vi "Trial - Editor.vi"(8 "Error IN":errorcluster) -> (0 "error out":errorcluster)   [LabVIEW 2018]
doc: "This VI allows the user to reprocess and reprint data sheets from previously run ESS test. User can search for vibe or thermal test for both actuators and controllers through this portal. Double click serial number from 'Available Data Files' listbox and press 'Print' to initiate report regeneration."
uses:
  controls/Trial Config Settings.ctl
  controls/Command IN_Recipe.ctl
  Globals/Global - Configuration Options.vi
panel:
  in  "Copy":bool
  in  "Trial Config Parameter Guide":bool
  in  "Rename":bool
  in  "Exit":bool
  out "Trial Name":string
  in  "Trial Settings":T1
  in  "Save":bool
  in  "New":bool
  in  "Delete":bool
  in  "Trial List":i32(listbox)
  in  "Refresh":bool
  out "Trial File Path":path
  in  "Functions":enum16{"Initialize", "Exit"}(ring)
  out "Trial Config Directory":path=path "C:/Data"
  # "Trial Configuration Screen"
  # "*click on trial file to view"
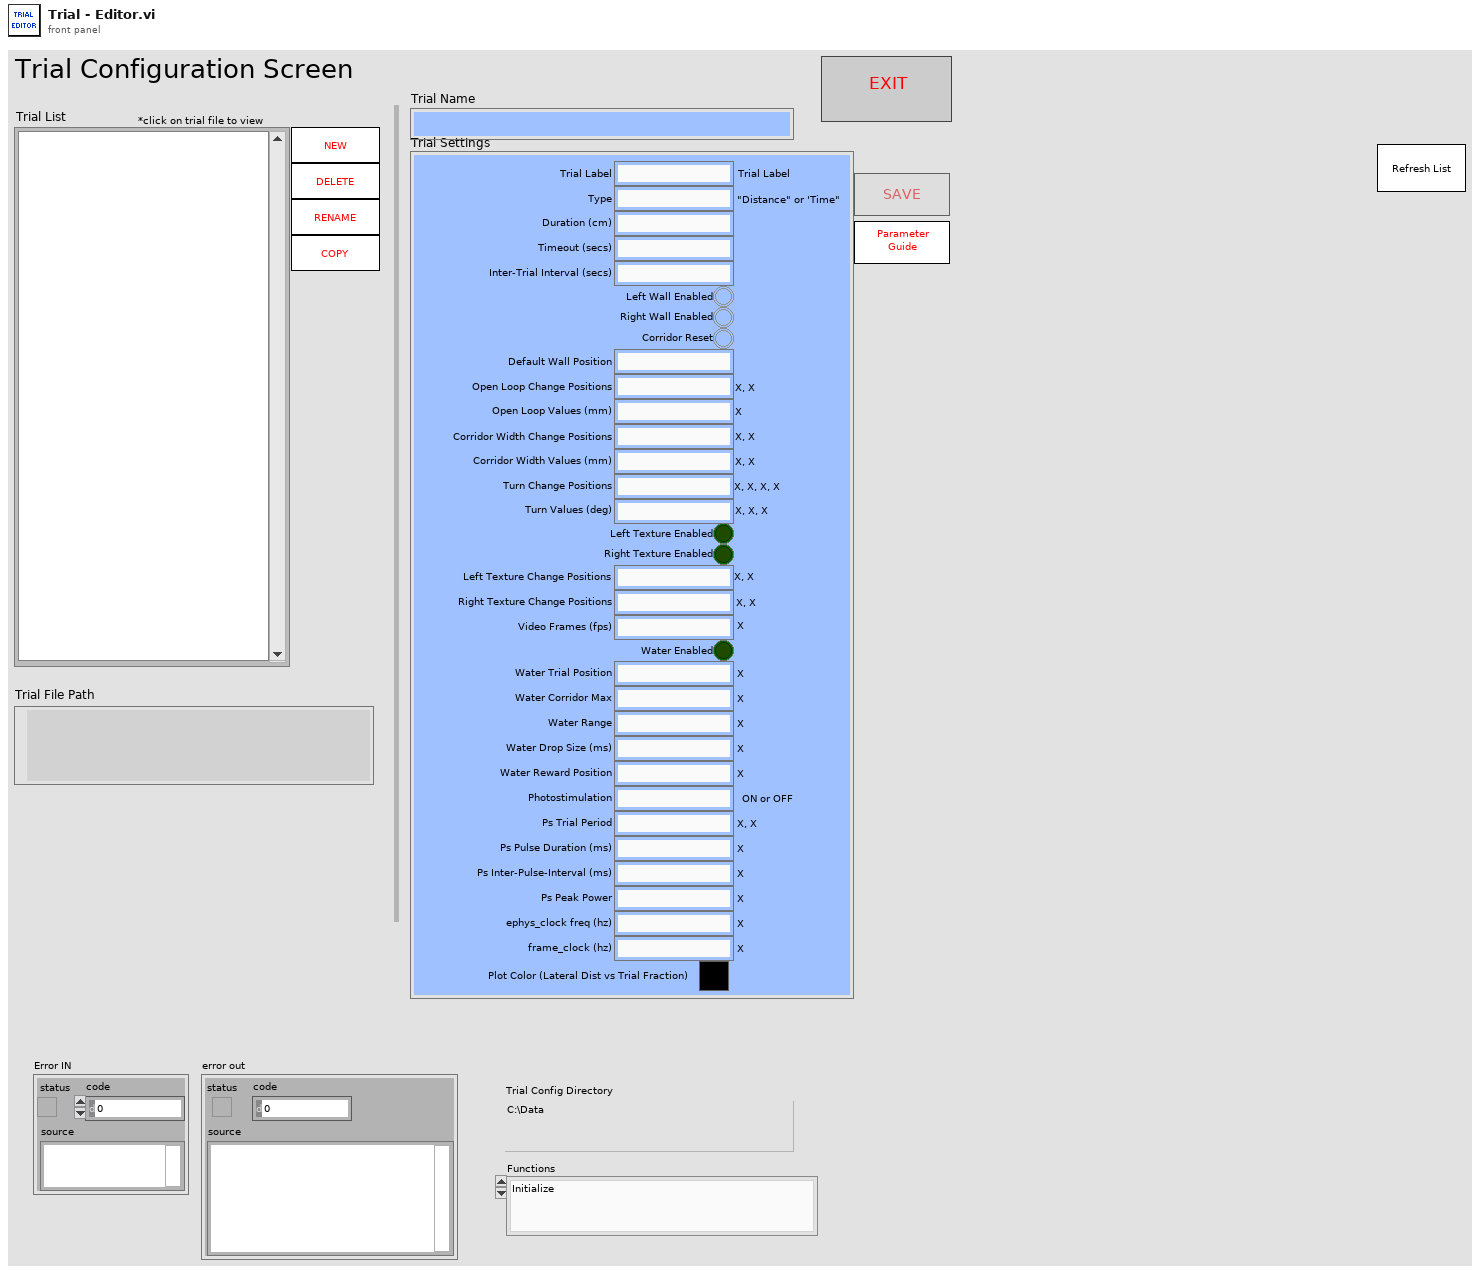
[diagram p1: front panel]
types:
  T1 = typedef "Trial Config Settings.ctl" = cluster{"Trial Label":string, "Type":string, "Timeout (secs)":string, "Inter-Trial Interval (secs)":string, "Left Wall Enabled":bool, "Right Wall Enabled":bool, "Corridor Reset":bool, "Default Wall Position":string, "Open Loop Change Positions":string, "Open Loop Values (mm)":string, "Corridor Width Change Positions":string, "Corridor Width Values (mm) ":string, "Turn Change Positions":string, "Turn Values (deg)":string, "Left Texture Change Positions":string, "Right Texture Change Positions":string, "Video Frames (fps)":string, "Water Enabled":bool, "Water Trial Position":string, "Photostimulation":string, "Water Corridor Max":string, "Water Range":string, "Water Drop Size (ms)":string, "Water Reward Position":string, "Duration (cm)":string, "Left Texture Enabled":bool, "Right Texture Enabled":bool, "Ps Trial Period":string, "Ps Inter-Pulse-Interval (ms)":string, "Ps Peak Power":string, "Ps Pulse Duration (ms)":string, "ephys_clock freq (hz)":string, "frame_clock (hz)":string, "Plot Color (Lateral Dist vs Trial Fraction)":u32}
  T2 = enum8{"Enabled", "Disabled", "Disabled and Grayed Out"}
  T3 = typedef "Command IN_Recipe.ctl" = enum16{"Save", "Load"}
  T4 = typedef "Rig Config Settings.ctl" = cluster{"Rig Name":string, "Rig Room":string, "Base Directory":string, "Computer IP Address":string, "Globals Name":string, "Treatmill Str":string, "cRIO Test Data Dir":path, "ai":string, "ao":string, "dio":string, "A_calib_str_row1":string, "A_calib_str_row2":string, "A_calib_str_row3":string, "Zero_V_str":string, "step_V":string, "Sample Freq":string, "ai_threshold":string, "run_speed_thresh":string, "speed_time_length":string, "wall ball gain":string, "max wall pos":string, "max cor width":string, "Trial Config Directory":path, "Randomize Trials?":bool}
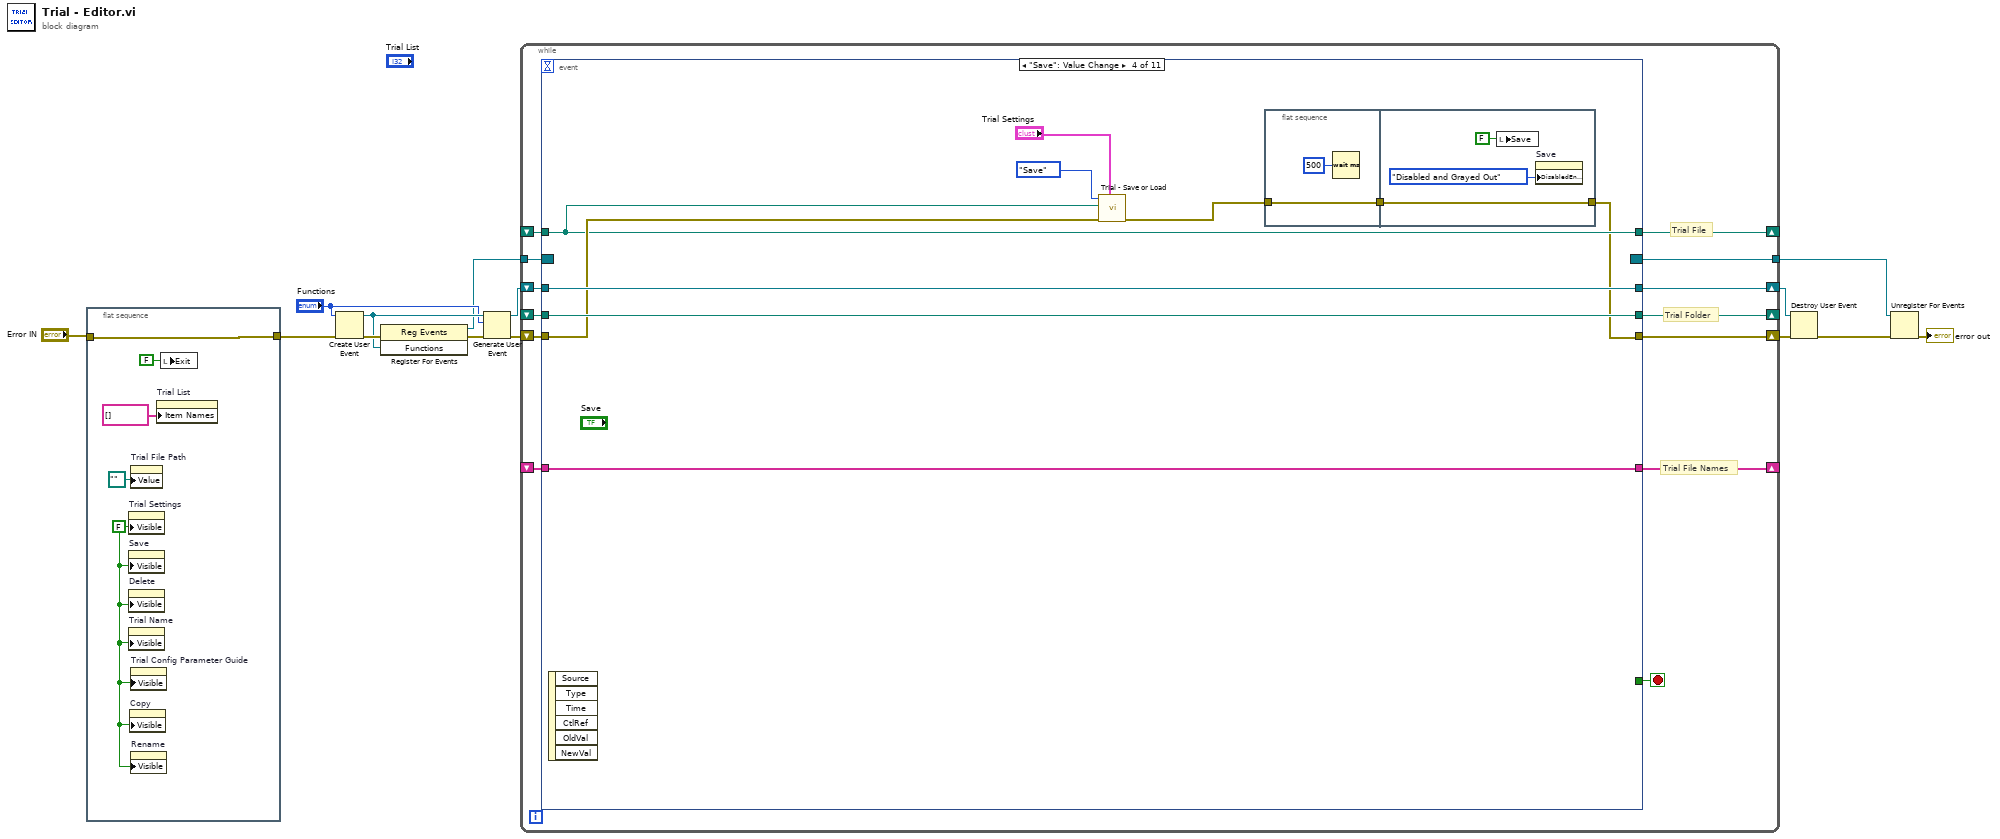
[diagram p0: block diagram]
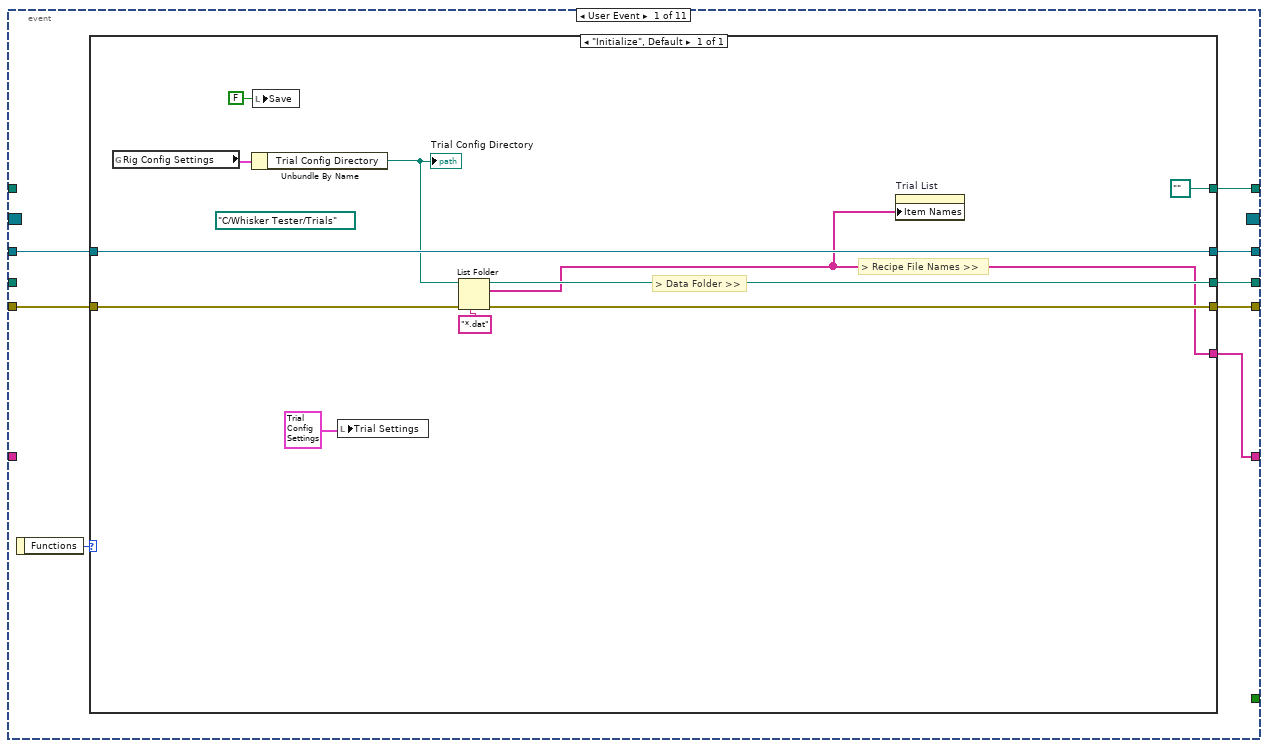
[diagram p2: hidden frame]
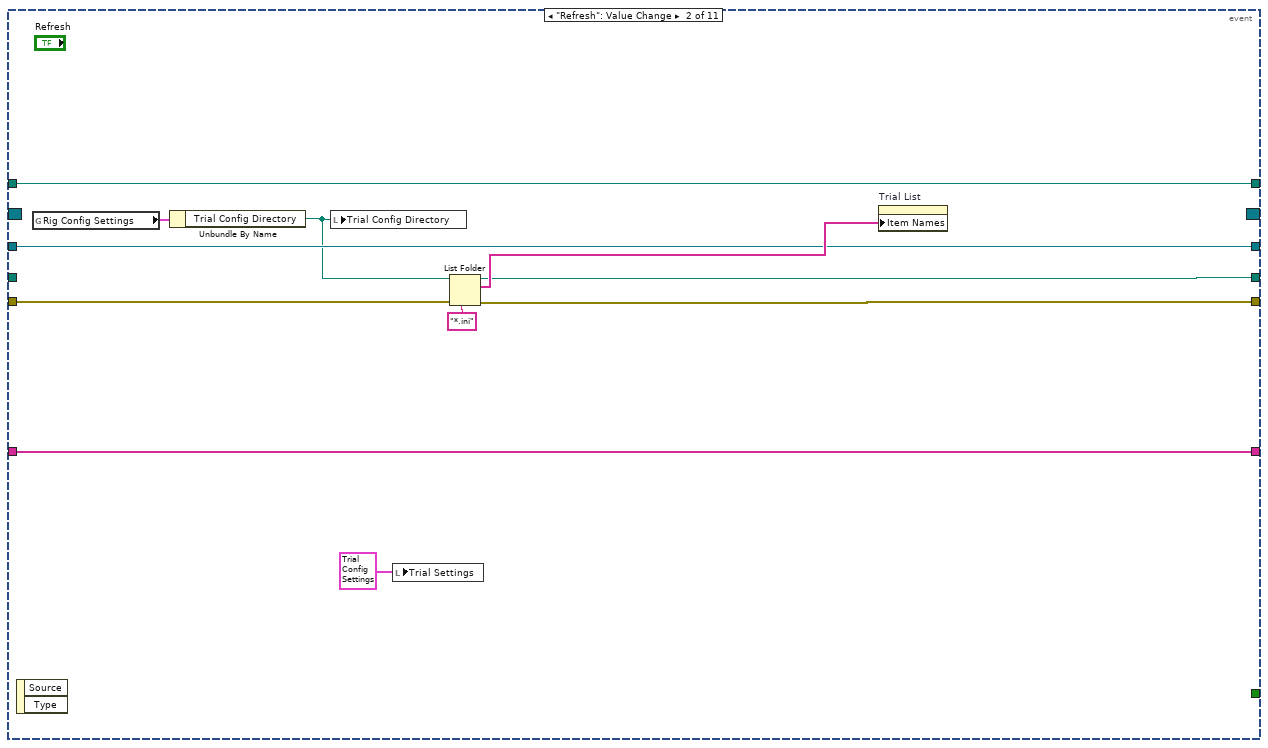
[diagram p3: hidden frame]
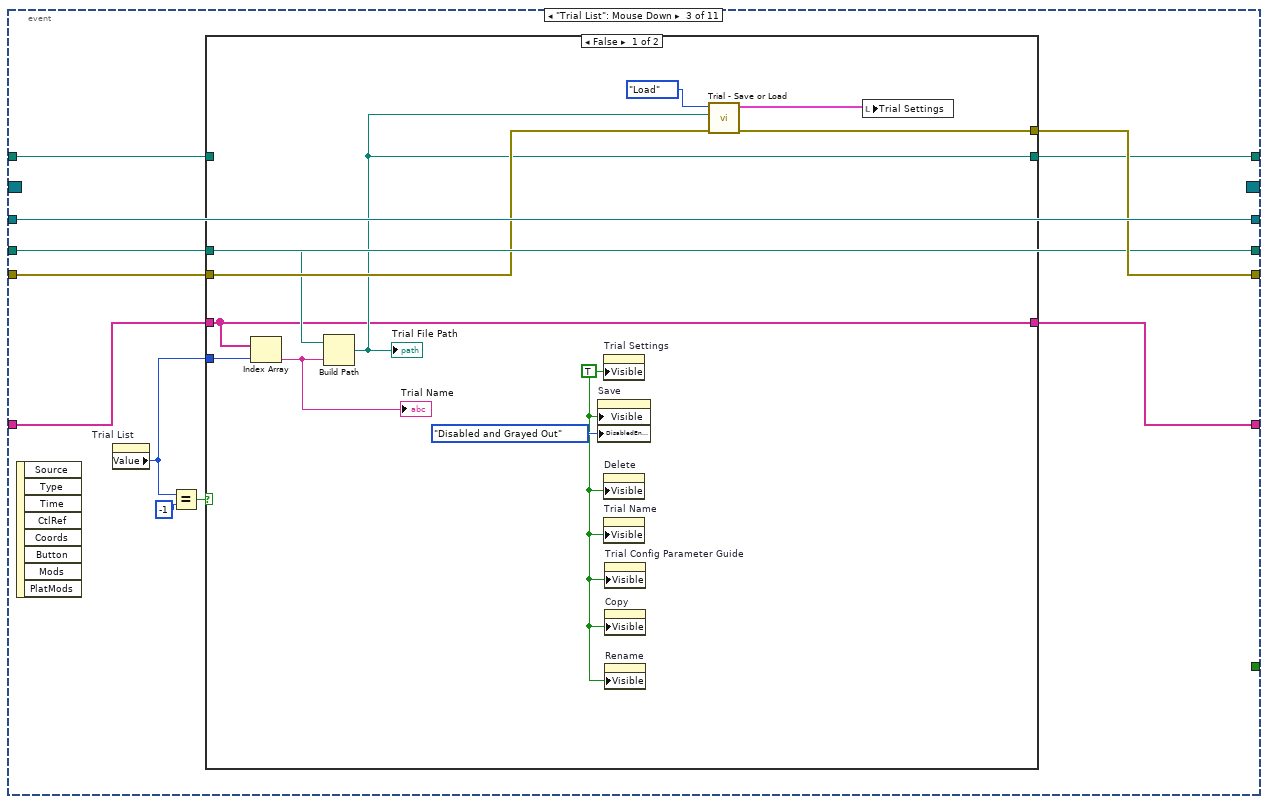
[diagram p4: hidden frame]
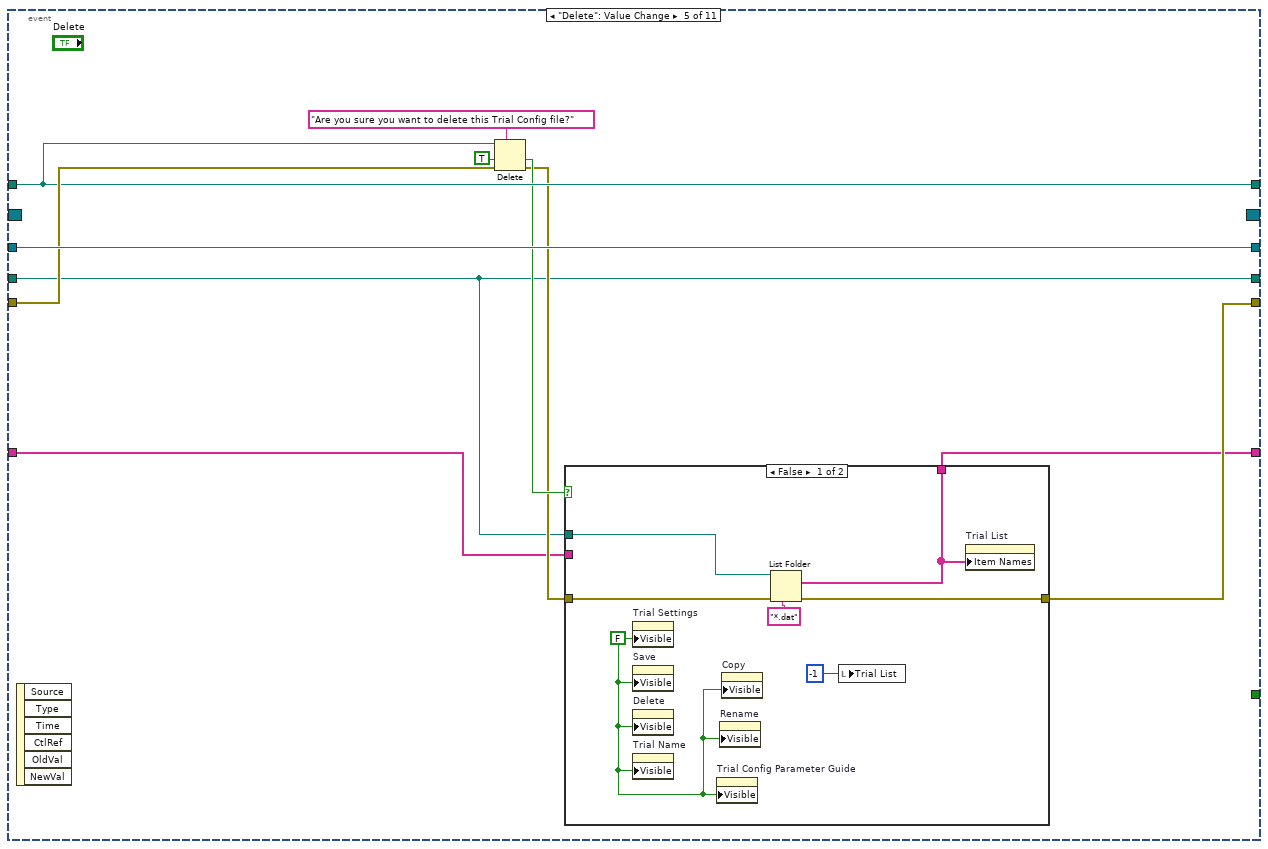
[diagram p6: hidden frame]
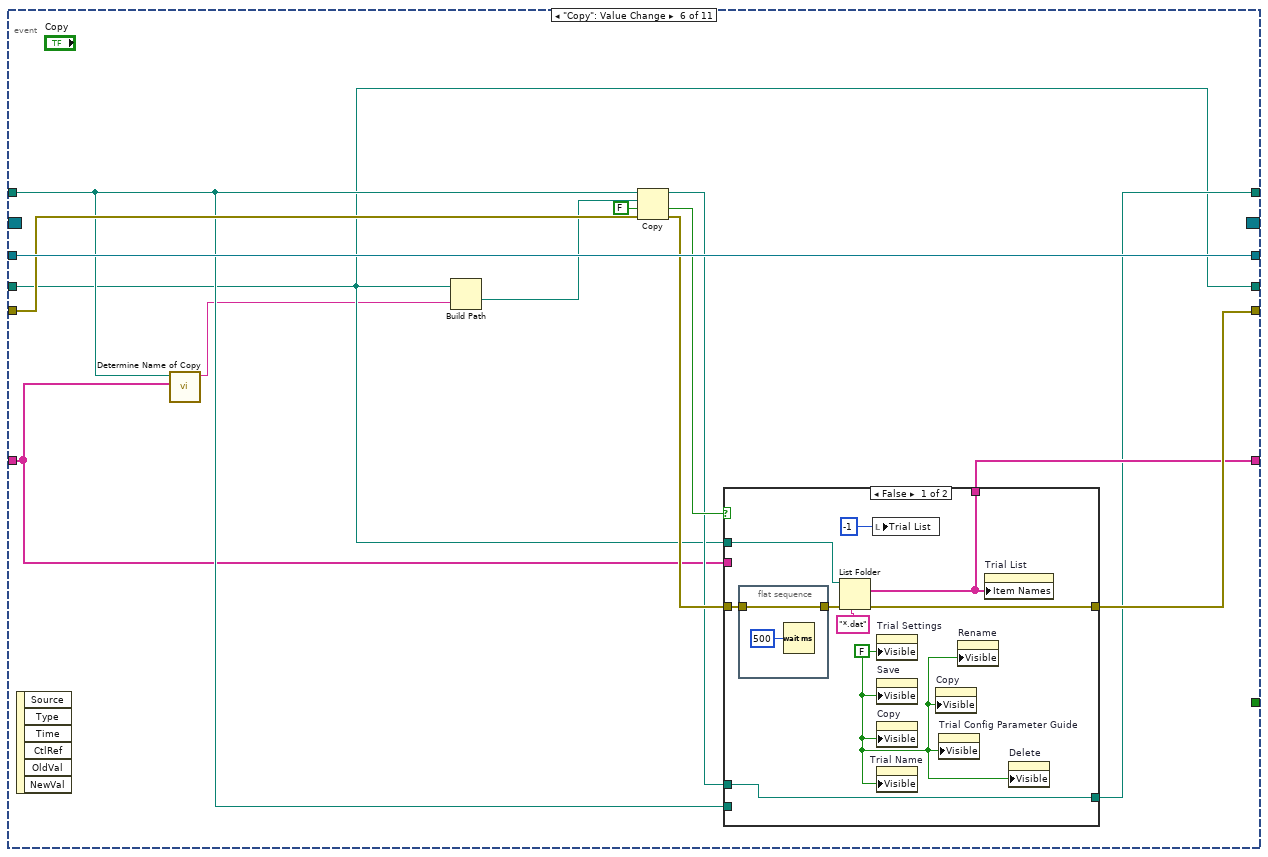
[diagram p8: hidden frame]
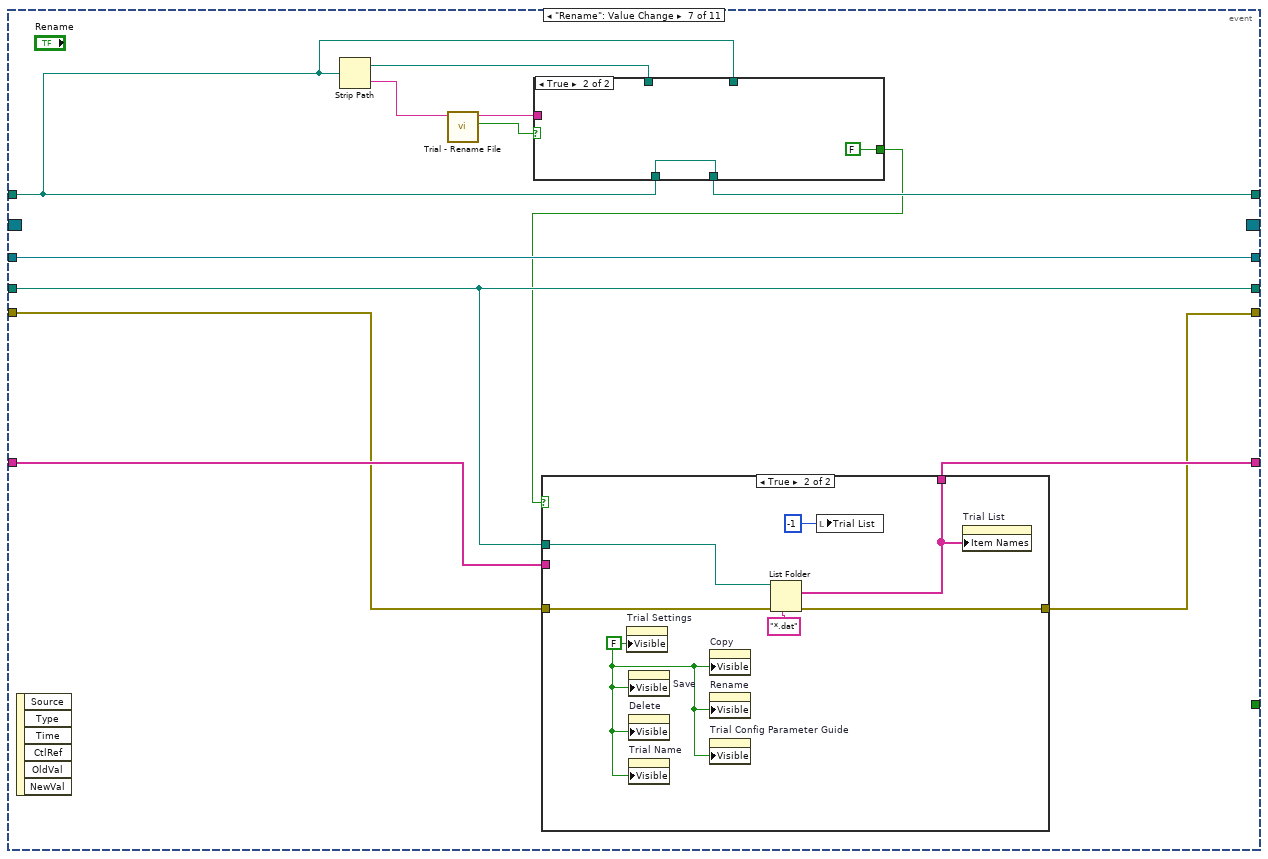
[diagram p10: hidden frame]
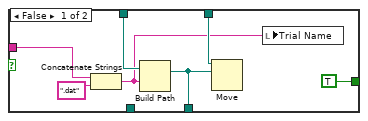
[diagram p11: hidden frame]
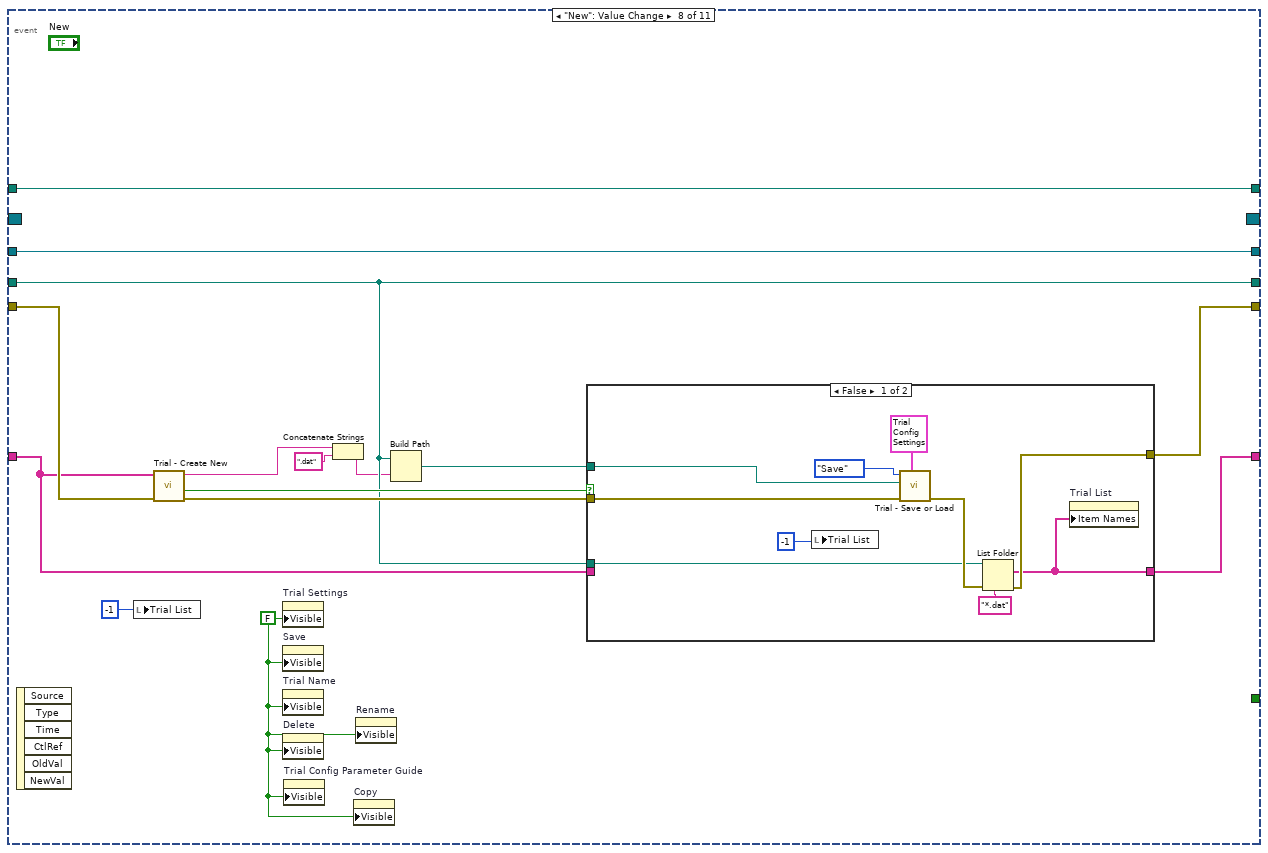
[diagram p13: hidden frame]
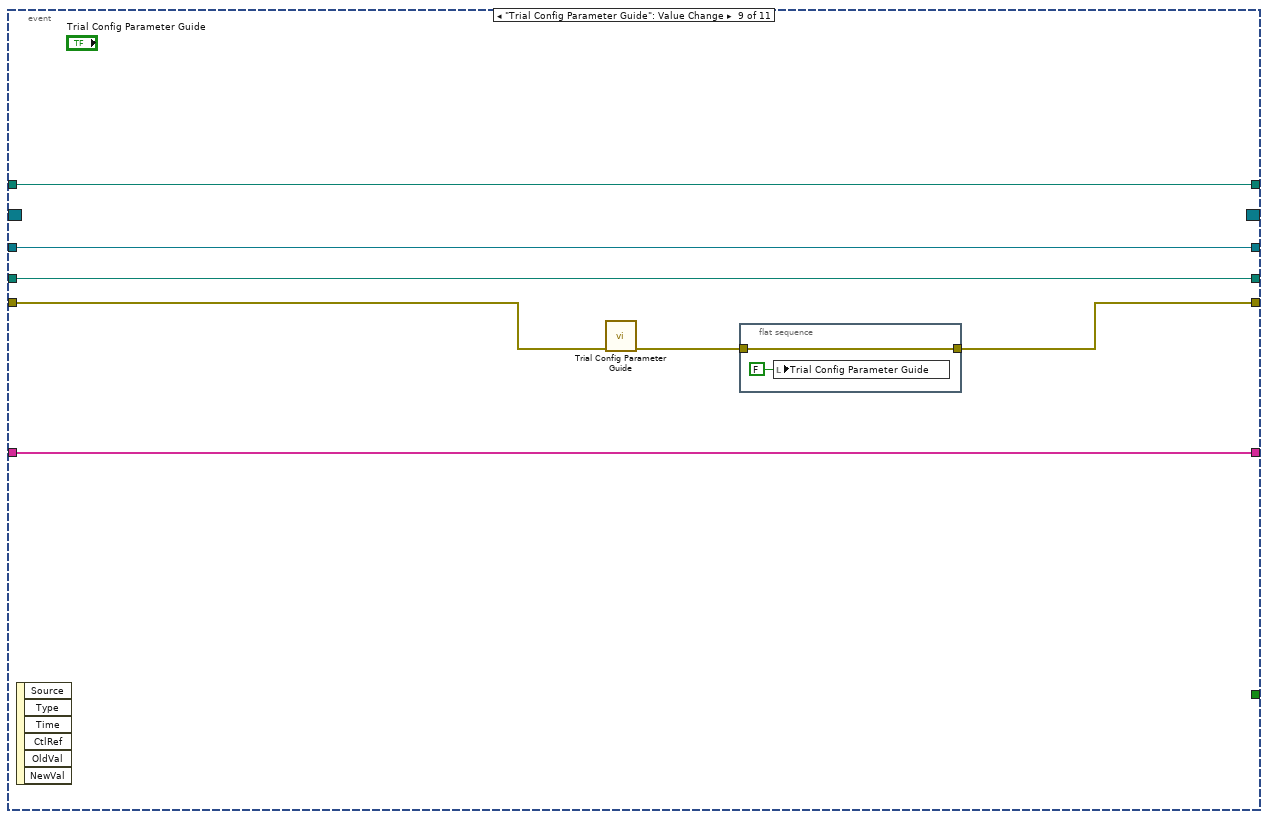
[diagram p15: hidden frame]
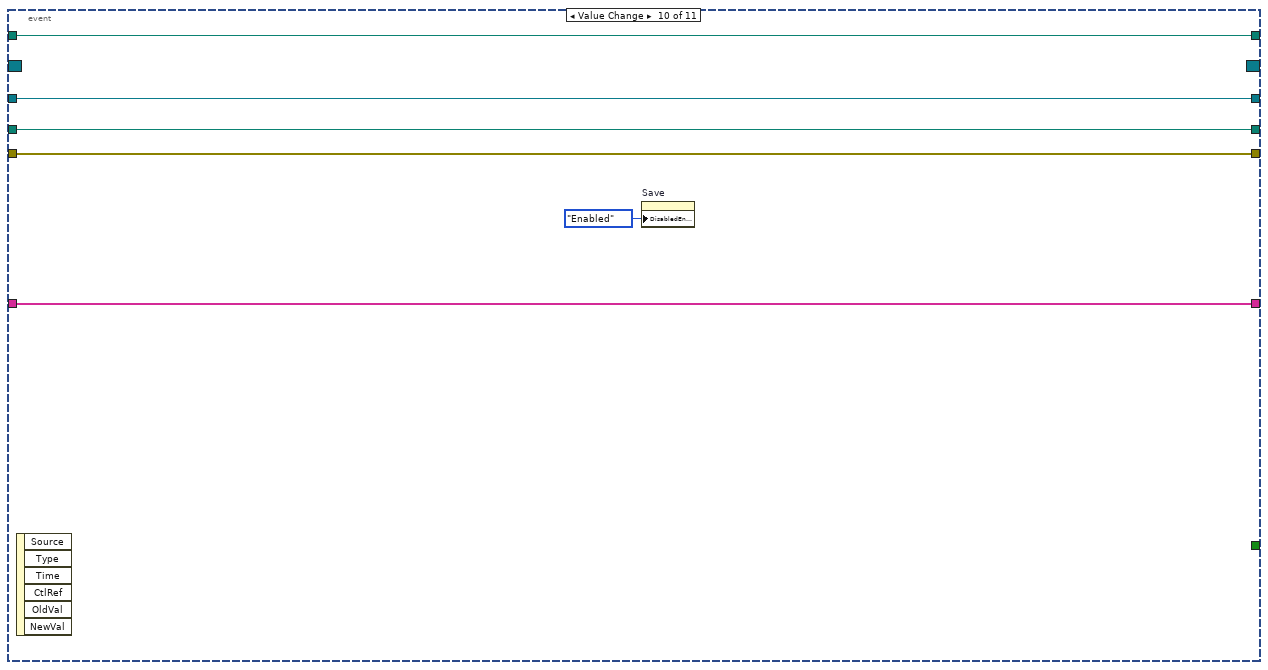
[diagram p16: hidden frame]
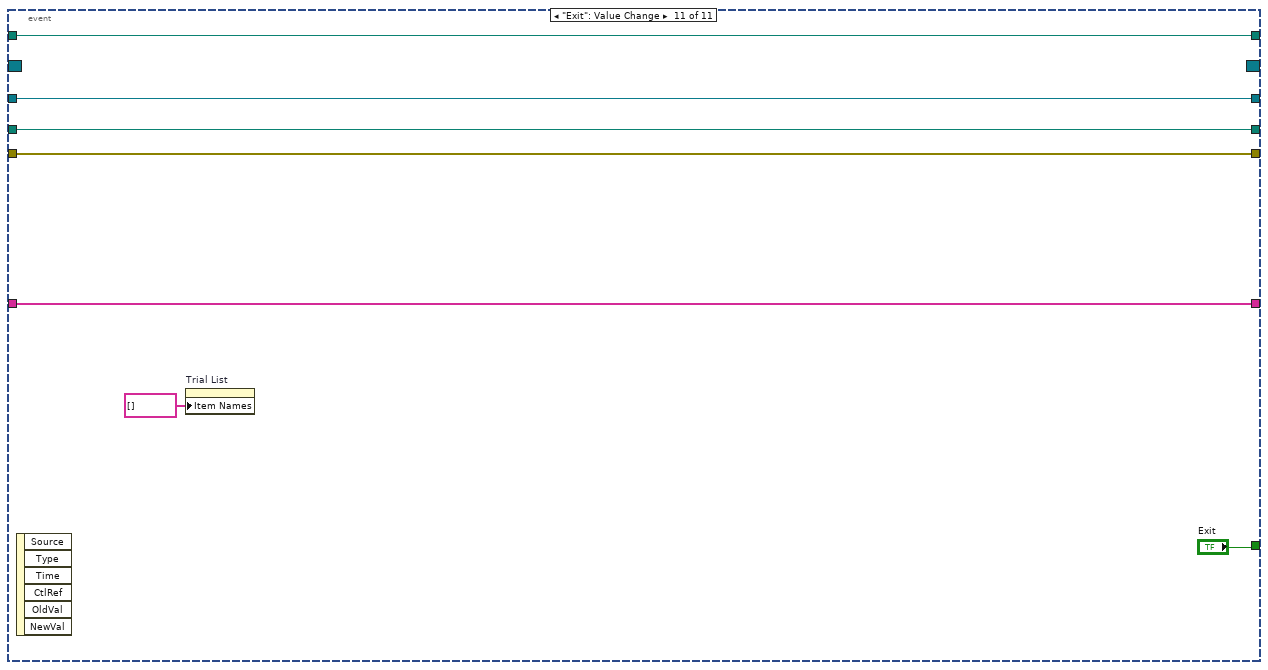
[diagram p17: hidden frame]
diagram:
  n1 = flat-sequence {
    tunnel: "Error IN" -> [w16]
    tunnel: [w16] -> w1
    frame #0 {
      w15 = FALSE ("Visible")
      n2 = property on="Trial Settings" class="Clust (strict)"("Visible"=w15) -> ()  [unwired: 2 in, 2 out]
      n3 = property on="Save" class="Bool (strict)"("Visible"=w15) -> ()  [unwired: 2 in, 2 out]
      n4 = property on="Delete" class="Bool"("Visible"=w15) -> ()  [unwired: 2 in, 2 out]
      n5 = property on="Trial Name" class="Str"("Visible"=w15) -> ()  [unwired: 2 in, 2 out]
      n6 = property on="Copy" class="Bool"("Visible"=w15) -> ()  [unwired: 2 in, 2 out]
      n7 = property on="Trial File Path" class="Path"("Value"=path "" ("Data File Selected")) -> ()  [unwired: 2 in, 2 out]
      n8 = property on="Trial Config Parameter Guide" class="Bool (strict)"("Visible"=w15) -> ()  [unwired: 2 in, 2 out]
      n9 = property on="Rename" class="Bool"("Visible"=w15) -> ()  [unwired: 2 in, 2 out]
      n10 = property on="Trial List" class="LstBox (strict)"("Item Names"=string[] []) -> ()  [unwired: 2 in, 2 out]
      n11 = local write "Exit"(FALSE ("Exit")) -> ()
    }
  }
  n12 = Create User Event(user event datatype="Functions", error in=w1) -> (user event=w12:refnum<user-event>, error out=w14:errorcluster)
  n13 = register-events(error in=w14, w12) -> (reference out=w10:refnum<event-registration>, error out=w13:errorcluster)  [unwired: 1 in]
  n14 = Generate User Event(user event=w12, event data cluster="Functions", error in=w13) -> (user event out=w8:refnum<user-event>, error out=w9:errorcluster)  [unwired: 1 in]
  n15 = while {
    tunnel: w10 -> [w32]
    shift-right: [w30] -> w7
    shift-left: w9 -> [w31]
    shift-right: [w29] -> _
    shift-left: _ -> [w23]
    shift-right: [w28] -> w6
    shift-left: w8 -> [w27]
    tunnel: [w26] -> w4
    shift-right: [w25] -> _
    shift-left: _ -> [w24]
    shift-right: [w21] -> _
    shift-left: _ -> [w20]
    stop <- w22 stop-if-true
    # "Trial File"
    # "Trial Folder"
    # "Trial File Names"
    n16 = event shown="[3] \"Save\": Value Change" {
      selector: w32 -> [_ _ _ _ _ _ _ _ _ _ _]
      dyn-events: [_ _ _ _ _ _ _ _ _ _ _] -> w26
      timeout: _ -> [_ _ _ _ _ _ _ _ _ _ _]
      tunnel: w31 -> [w39 w59 w71 w94 w112 w133 w152 w194 w211 w220 w228]
      tunnel: [w38 w58 w70 w91 w107 w135 w151 w191 w209 w220 w228] -> w30
      tunnel: [w37 w57 w69 w95 w104 w127 w160 w189 w213 w221 w227] -> w29
      tunnel: [w36 w56 w72 w96 w113 w136 w163 w196 w214 w222 w229] -> w28
      tunnel: w27 -> [w35 w56 w72 w96 w113 w136 w163 w196 w214 w222 w229]
      tunnel: [w34 w54 w63 w97 w106 w134 w162 w185 w212 w219 w226] -> w25
      tunnel: w24 -> [_ w54 w73 w97 w105 w126 w161 w183 w212 w219 w226]
      tunnel: w23 -> [_ _ w69 w95 w104 w127 w160 w189 w213 w221 w227]
      tunnel: [_ _ _ _ _ _ _ _ _ _ "Exit"] -> w22
      tunnel: [w33 w62 w68 w93 w111 w130 w154 w195 w215 w223 w230] -> w21
      tunnel: w20 -> [_ w62 w64 w93 w111 w128 w155 w195 w215 w223 w230]
      event User Event {
        n17 = event-data() -> ("Functions"=w40:enum16{"Initialize", "Exit"})  [unwired: 1 in]
        n18 = case shown="\"Initialize\", Default" w40 {
          tunnel: w39 -> [w50]
          tunnel: [w49] -> w38
          tunnel: [w48] -> w37
          tunnel: [w47] -> w36
          tunnel: w35 -> [w47]
          tunnel: [w43] -> w34
          tunnel: [path "" ("appended path")] -> w33
          frame "Initialize", Default {
            (unwired) path "C:/Whisker Tester/Trials" ("path")
            # "> Recipe File Names >>"
            # "> Data Folder >>"
            n19 = global read "Global - Configuration Options.vi" "Rig Config Settings"() -> (w45:T4)
            n20 = Unbundle By Name(w45) -> ("Trial Config Directory"=w41:path)
            "Trial Config Directory" <- w41
            n21 = local write "Save"(FALSE ("Save")) -> ()
            n22 = local write "Trial Settings"(T1 {"Trial Label"="", "Type"="", "Timeout (secs)"="", "Inter-Trial Interval (secs)"="", "Left Wall Enabled"=FALSE, "Right Wall Enabled"=FALSE, "Corridor Reset"=FALSE, "Default Wall Position"="", "Open Loop Change Positions"="", "Open Loop Values (mm)"="", "Corridor Width Change Positions"="", "Corridor Width Values (mm) "="", "Turn Change Positions"="0", "Turn Values (deg)"="", "Left Texture Change Positions"="", "Right Texture Change Positions"="", "Video Frames (fps)"="", "Water Enabled"=FALSE, "Water Trial Position"="", "Photostimulation"="", "Water Corridor Max"="", "Water Range"="", "Water Drop Size (ms)"="", "Water Reward Position"="", "Duration (cm)"="", "Left Texture Enabled"=FALSE, "Right Texture Enabled"=FALSE, "Ps Trial Period"="", "Ps Inter-Pulse-Interval (ms)"="", "Ps Peak Power"="", "Ps Pulse Duration (ms)"="", "ephys_clock freq (hz)"="", "frame_clock (hz)"="", "Plot Color (Lateral Dist vs Trial Fraction)"=0} ("Part Recipe Settings IN")) -> ()
            n23 = List Folder(path=w41, pattern="*.dat", error in=w50) -> (path out=w48:path, filenames=w43:string[], error out=w49:errorcluster)  [unwired: 1 in, 1 out]
            n24 = property on="Trial List" class="LstBox (strict)"("Item Names"=w43) -> ()  [unwired: 2 in, 2 out]
          }
        }
      }
      event "Refresh": Value Change {
        n25 = event-data() -> ()  [unwired: 1 in, 2 out]
        n26 = global read "Global - Configuration Options.vi" "Rig Config Settings"() -> (w52:T4)
        n27 = Unbundle By Name(w52) -> ("Trial Config Directory"=w55:path)
        n28 = local write "Trial Config Directory"(w55) -> ()
        n29 = local write "Trial Settings"(T1 {"Trial Label"="", "Type"="", "Timeout (secs)"="", "Inter-Trial Interval (secs)"="", "Left Wall Enabled"=FALSE, "Right Wall Enabled"=FALSE, "Corridor Reset"=FALSE, "Default Wall Position"="", "Open Loop Change Positions"="", "Open Loop Values (mm)"="", "Corridor Width Change Positions"="", "Corridor Width Values (mm) "="", "Turn Change Positions"="0", "Turn Values (deg)"="", "Left Texture Change Positions"="", "Right Texture Change Positions"="", "Video Frames (fps)"="", "Water Enabled"=FALSE, "Water Trial Position"="", "Photostimulation"="", "Water Corridor Max"="", "Water Range"="", "Water Drop Size (ms)"="", "Water Reward Position"="", "Duration (cm)"="", "Left Texture Enabled"=FALSE, "Right Texture Enabled"=FALSE, "Ps Trial Period"="", "Ps Inter-Pulse-Interval (ms)"="", "Ps Peak Power"="", "Ps Pulse Duration (ms)"="", "ephys_clock freq (hz)"="", "frame_clock (hz)"="", "Plot Color (Lateral Dist vs Trial Fraction)"=0} ("Part Recipe Settings IN")) -> ()
        n30 = List Folder(path=w55, pattern="*.ini", error in=w59) -> (path out=w57:path, filenames=w60:string[], error out=w58:errorcluster)  [unwired: 1 in, 1 out]
        n31 = property on="Trial List" class="LstBox (strict)"("Item Names"=w60) -> ()  [unwired: 2 in, 2 out]
      }
      event "Trial List": Mouse Down {
        n32 = event-data() -> ()  [unwired: 1 in, 8 out]
        n33 = property on="Trial List" class="LstBox (strict)"() -> ("Value"=w66:i32)  [unwired: 2 in, 2 out]
        n34 = Equal?(x=w66, y=-1) -> (x = y?=w67:bool)
        n35 = case shown="False" w67 {
          tunnel: w73 -> [w77 w85]
          tunnel: w71 -> [w84 w87]
          tunnel: [w83 w87] -> w70
          tunnel: w69 -> [w82 _]
          tunnel: [w80 w86] -> w68
          tunnel: w66 -> [w78 _]
          tunnel: w64 -> [_ w86]
          tunnel: [w77 w85] -> w63
          frame False {
            w74 = TRUE ("Visible")
            n36 = Index Array(array=w77, index=w78) -> (element=w81:string)
            "Trial Name" <- w81
            n37 = Build Path(base path=w82, name or relative path=w81) -> (appended path=w80:path)
            "Trial File Path" <- w80
            n38 = property on="Save" class="Bool (strict)"("Visible"=w74, "DisabledEnum"=T2."Disabled and Grayed Out" ("Disabled")) -> ()  [unwired: 2 in, 2 out]
            n39 = property on="Trial Settings" class="Clust (strict)"("Visible"=w74) -> ()  [unwired: 2 in, 2 out]
            n40 = property on="Delete" class="Bool"("Visible"=w74) -> ()  [unwired: 2 in, 2 out]
            n41 = property on="Trial Name" class="Str"("Visible"=w74) -> ()  [unwired: 2 in, 2 out]
            n42 = property on="Trial Config Parameter Guide" class="Bool (strict)"("Visible"=w74) -> ()  [unwired: 2 in, 2 out]
            n43 = property on="Copy" class="Bool"("Visible"=w74) -> ()  [unwired: 2 in, 2 out]
            n44 = property on="Rename" class="Bool"("Visible"=w74) -> ()  [unwired: 2 in, 2 out]
            n45 = call "Trial - Save or Load.vi"("Error IN"=w84, "Trial Path IN"=w80, "Command IN"=Command_IN_Recipe."Load") -> ("Error OUT"=w83:errorcluster, "Trial Settings OUT"=w79:T1)  [unwired: 7 in]
            n46 = local write "Trial Settings"(w79) -> ()
          }
          frame True {
          }
        }
      }
      event "Save": Value Change {
        n47 = event-data() -> ()  [unwired: 1 in, 6 out]
        n48 = call "Trial - Save or Load.vi"("Trial Settings IN"="Trial Settings", "Error IN"=w94, "Trial Path IN"=w93, "Command IN"=Command_IN_Recipe."Save") -> ("Error OUT"=w92:errorcluster)  [unwired: 6 in, 1 out]
        n49 = flat-sequence {
          tunnel: w92 -> [w99]
          tunnel: [w99] -> w90
          tunnel: [w102] -> w91
          tunnel: w90 -> [w102]
          frame #0 {
            n50 = Wait (ms)(milliseconds to wait=u32 500) -> ()  [unwired: 1 out]
          }
          frame #1 {
            n51 = local write "Save"(FALSE ("Save")) -> ()
            n52 = property on="Save" class="Bool (strict)"("DisabledEnum"=T2."Disabled and Grayed Out" ("Disabled")) -> ()  [unwired: 2 in, 2 out]
          }
        }
      }
      event "Delete": Value Change {
        n53 = event-data() -> ()  [unwired: 1 in, 6 out]
        n54 = Delete(prompt (Delete)="Are you sure you want to delete this Trial Config file?", path (use dialog)=w111, confirm (F)=TRUE, error in=w112) -> (cancelled=w109:bool, error out=w108:errorcluster)  [unwired: 1 in, 1 out]
        n55 = case shown="False" w109 {
          tunnel: w108 -> [w119 w122]
          tunnel: [w118 w122] -> w107
          tunnel: [w117 w121] -> w106
          tunnel: w105 -> [_ w121]
          tunnel: w104 -> [w116 _]
          frame False {
            w114 = FALSE ("Visible")
            n56 = property on="Trial Settings" class="Clust (strict)"("Visible"=w114) -> ()  [unwired: 2 in, 2 out]
            n57 = property on="Save" class="Bool (strict)"("Visible"=w114) -> ()  [unwired: 2 in, 2 out]
            n58 = property on="Delete" class="Bool"("Visible"=w114) -> ()  [unwired: 2 in, 2 out]
            n59 = property on="Trial Name" class="Str"("Visible"=w114) -> ()  [unwired: 2 in, 2 out]
            n60 = property on="Trial Config Parameter Guide" class="Bool (strict)"("Visible"=w114) -> ()  [unwired: 2 in, 2 out]
            n61 = property on="Rename" class="Bool"("Visible"=w114) -> ()  [unwired: 2 in, 2 out]
            n62 = property on="Copy" class="Bool"("Visible"=w114) -> ()  [unwired: 2 in, 2 out]
            n63 = List Folder(path=w116, pattern="*.dat", error in=w119) -> (filenames=w117:string[], error out=w118:errorcluster)  [unwired: 1 in, 2 out]
            n64 = local write "Trial List"(-1 ("Recipe List")) -> ()
            n65 = property on="Trial List" class="LstBox (strict)"("Item Names"=w117) -> ()  [unwired: 2 in, 2 out]
          }
          frame True {
          }
        }
      }
      event "Copy": Value Change {
        n66 = event-data() -> ()  [unwired: 1 in, 6 out]
        n67 = call "Determine Name of Copy.vi"("All Trial Files"=w126, "Trial File Path"=w128) -> ("Name of Copy"=w125:string)  [unwired: 9 in]
        n68 = Build Path(base path=w127, name or relative path=w125) -> (appended path=w123:path)
        n69 = Copy(8:w133, 9:FALSE ("overwrite (F)"), 10:w123, 11:w128) -> (0:w132:errorcluster, 1:w131:bool, 3:w129:path)  [unwired: 1 in]
        n70 = case shown="False" w131 {
          tunnel: w132 -> [w139 w150]
          tunnel: [w144 w150] -> w135
          tunnel: [w143 w149] -> w134
          tunnel: w126 -> [_ w149]
          tunnel: w127 -> [w142 _]
          tunnel: [w140 w148] -> w130
          tunnel: w128 -> [_ w148]
          tunnel: w129 -> [w140 _]
          frame False {
            w137 = FALSE ("Visible")
            n71 = flat-sequence {
              tunnel: w139 -> [w147]
              tunnel: [w147] -> w138
              frame #0 {
                n72 = Wait (ms)(milliseconds to wait=u32 500) -> ()  [unwired: 1 out]
              }
            }
            n73 = List Folder(path=w142, pattern="*.dat", error in=w138) -> (filenames=w143:string[], error out=w144:errorcluster)  [unwired: 1 in, 2 out]
            n74 = local write "Trial List"(-1 ("Recipe List")) -> ()
            n75 = property on="Trial Settings" class="Clust (strict)"("Visible"=w137) -> ()  [unwired: 2 in, 2 out]
            n76 = property on="Save" class="Bool (strict)"("Visible"=w137) -> ()  [unwired: 2 in, 2 out]
            n77 = property on="Copy" class="Bool"("Visible"=w137) -> ()  [unwired: 2 in, 2 out]
            n78 = property on="Trial Name" class="Str"("Visible"=w137) -> ()  [unwired: 2 in, 2 out]
            n79 = property on="Copy" class="Bool"("Visible"=w137) -> ()  [unwired: 2 in, 2 out]
            n80 = property on="Trial Config Parameter Guide" class="Bool (strict)"("Visible"=w137) -> ()  [unwired: 2 in, 2 out]
            n81 = property on="Rename" class="Bool"("Visible"=w137) -> ()  [unwired: 2 in, 2 out]
            n82 = property on="Trial List" class="LstBox (strict)"("Item Names"=w143) -> ()  [unwired: 2 in, 2 out]
            n83 = property on="Delete" class="Bool"("Visible"=w137) -> ()  [unwired: 2 in, 2 out]
          }
          frame True {
          }
        }
      }
      event "Rename": Value Change {
        n84 = event-data() -> ()  [unwired: 1 in, 6 out]
        n85 = Strip Path(path=w155) -> (stripped path=w159:path, name=w158:string)
        n86 = call "Trial - Rename File.vi"("Current File Name"=w158) -> ("Cancel OUT"=w156:bool, "Enter New File Name OUT"=w157:string)  [unwired: 9 in]
        n87 = case shown="True" w156 {
          tunnel: w159 -> [w169 _]
          tunnel: w155 -> [w168 _]
          tunnel: w157 -> [w167 _]
          tunnel: w155 -> [_ w172]
          tunnel: [w166 w172] -> w154
          tunnel: [TRUE FALSE] -> w153
          frame False {
            n88 = Concatenate Strings(w167, ".dat") -> (w164:string)
            n89 = Build Path(base path=w169, name or relative path=w164) -> (appended path=w166:path)
            n90 = Move(source path=w168, 10:w166) -> ()  [unwired: 3 in, 3 out]
            n91 = local write "Trial Name"(w164) -> ()
          }
          frame True {
          }
        }
        n92 = case shown="True" w153 {
          tunnel: w152 -> [w174 w180]
          tunnel: [w174 w179] -> w151
          tunnel: [w173 w178] -> w162
          tunnel: w161 -> [w173 _]
          tunnel: w160 -> [_ w177]
          frame False {
          }
          frame True {
            w175 = FALSE ("Visible")
            n93 = property on="Trial Settings" class="Clust (strict)"("Visible"=w175) -> ()  [unwired: 2 in, 2 out]
            n94 = property on="Save" class="Bool (strict)"("Visible"=w175) -> ()  [unwired: 2 in, 2 out]
            n95 = property on="Delete" class="Bool"("Visible"=w175) -> ()  [unwired: 2 in, 2 out]
            n96 = property on="Trial Name" class="Str"("Visible"=w175) -> ()  [unwired: 2 in, 2 out]
            n97 = property on="Copy" class="Bool"("Visible"=w175) -> ()  [unwired: 2 in, 2 out]
            n98 = property on="Rename" class="Bool"("Visible"=w175) -> ()  [unwired: 2 in, 2 out]
            n99 = property on="Trial Config Parameter Guide" class="Bool (strict)"("Visible"=w175) -> ()  [unwired: 2 in, 2 out]
            n100 = List Folder(path=w177, pattern="*.dat", error in=w180) -> (filenames=w178:string[], error out=w179:errorcluster)  [unwired: 1 in, 2 out]
            n101 = local write "Trial List"(-1 ("Recipe List")) -> ()
            n102 = property on="Trial List" class="LstBox (strict)"("Item Names"=w178) -> ()  [unwired: 2 in, 2 out]
          }
        }
      }
      event "New": Value Change {
        w182 = FALSE ("Visible")
        n103 = event-data() -> ()  [unwired: 1 in, 6 out]
        n104 = local write "Trial List"(-1 ("Recipe List")) -> ()
        n105 = call "Trial - Create New.vi"("Error IN"=w194, "Existing Recipe Names"=w183) -> ("Error OUT"=w192:errorcluster, "Cancel OUT"=w193:bool, "Enter New Recipe File Name OUT"=w187:string)  [unwired: 7 in]
        n106 = property on="Trial Settings" class="Clust (strict)"("Visible"=w182) -> ()  [unwired: 2 in, 2 out]
        n107 = property on="Save" class="Bool (strict)"("Visible"=w182) -> ()  [unwired: 2 in, 2 out]
        n108 = property on="Trial Name" class="Str"("Visible"=w182) -> ()  [unwired: 2 in, 2 out]
        n109 = property on="Delete" class="Bool"("Visible"=w182) -> ()  [unwired: 2 in, 2 out]
        n110 = property on="Trial Config Parameter Guide" class="Bool (strict)"("Visible"=w182) -> ()  [unwired: 2 in, 2 out]
        n111 = Concatenate Strings(w187, ".dat" ("string")) -> (w186:string)
        n112 = property on="Copy" class="Bool"("Visible"=w182) -> ()  [unwired: 2 in, 2 out]
        n113 = property on="Rename" class="Bool"("Visible"=w182) -> ()  [unwired: 2 in, 2 out]
        n114 = Build Path(base path=w189, name or relative path=w186) -> (appended path=w190:path)
        n115 = case shown="False" w193 {
          tunnel: w192 -> [w206 w208]
          tunnel: [w201 w208] -> w191
          tunnel: w190 -> [w204 _]
          tunnel: w189 -> [w200 _]
          tunnel: [w199 w207] -> w185
          tunnel: w183 -> [_ w207]
          frame False {
            n116 = local write "Trial List"(-1 ("Recipe List")) -> ()
            n117 = call "Trial - Save or Load.vi"("Trial Settings IN"=T1 {"Trial Label"="", "Type"="", "Timeout (secs)"="", "Inter-Trial Interval (secs)"="", "Left Wall Enabled"=FALSE, "Right Wall Enabled"=FALSE, "Corridor Reset"=FALSE, "Default Wall Position"="", "Open Loop Change Positions"="", "Open Loop Values (mm)"="", "Corridor Width Change Positions"="", "Corridor Width Values (mm) "="", "Turn Change Positions"="0", "Turn Values (deg)"="", "Left Texture Change Positions"="", "Right Texture Change Positions"="", "Video Frames (fps)"="", "Water Enabled"=FALSE, "Water Trial Position"="", "Photostimulation"="", "Water Corridor Max"="", "Water Range"="", "Water Drop Size (ms)"="", "Water Reward Position"="", "Duration (cm)"="", "Left Texture Enabled"=FALSE, "Right Texture Enabled"=FALSE, "Ps Trial Period"="", "Ps Inter-Pulse-Interval (ms)"="", "Ps Peak Power"="", "Ps Pulse Duration (ms)"="", "ephys_clock freq (hz)"="", "frame_clock (hz)"="", "Plot Color (Lateral Dist vs Trial Fraction)"=0} ("Part Recipe Settings IN"), "Error IN"=w206, "Trial Path IN"=w204, "Command IN"=Command_IN_Recipe."Save") -> ("Error OUT"=w202:errorcluster)  [unwired: 6 in, 1 out]
            n118 = List Folder(path=w200, pattern="*.dat", error in=w202) -> (filenames=w199:string[], error out=w201:errorcluster)  [unwired: 1 in, 2 out]
            n119 = property on="Trial List" class="LstBox (strict)"("Item Names"=w199) -> ()  [unwired: 2 in, 2 out]
          }
          frame True {
          }
        }
      }
      event "Trial Config Parameter Guide": Value Change {
        n120 = event-data() -> ()  [unwired: 1 in, 6 out]
        n121 = call "Trial Config Parameter Guide.vi"("Error IN"=w211) -> ("Error OUT"=w210:errorcluster)  [unwired: 10 in]
        n122 = flat-sequence {
          tunnel: w210 -> [w216]
          tunnel: [w216] -> w209
          frame #0 {
            n123 = local write "Trial Config Parameter Guide"(FALSE ("Trial Config Parameter Guide")) -> ()
          }
        }
      }
      event Value Change {
        n124 = event-data() -> ()  [unwired: 1 in, 6 out]
        n125 = property on="Save" class="Bool (strict)"("DisabledEnum"=T2."Enabled" ("Disabled")) -> ()  [unwired: 2 in, 2 out]
      }
      event "Exit": Value Change {
        n126 = event-data() -> ()  [unwired: 1 in, 6 out]
        n127 = property on="Trial List" class="LstBox (strict)"("Item Names"=string[] []) -> ()  [unwired: 2 in, 2 out]
      }
    }
  }
  n128 = Destroy User Event(user event=w6, error in=w7) -> (error out=w5:errorcluster)
  n129 = Unregister For Events(event registration refnum=w4, error in=w5) -> (error out=→"error out":errorcluster)
